vi "RT Loop - Sequence Engine.vi"(8 "error in (no error)":errorcluster, 9 "FPGA VI Reference":T1, 10 "Message Queue":refnum<queue>, 11 "Sequence Queue":refnum<queue>) -> ()   [LabVIEW 2018]
doc: "Executes the sequence sent from the main UI."
uses:
  support/Message Queue/Message Cluster.ctl
  controls/Sequence Command.ctl
  controls/Sequence Engine State.ctl
  controls/FPGA VI Reference.ctl
  controls/Control Configuration.ctl
  Globals/Global - All RT Loop Stop.vi
  <vilib>/Utility/error.llb/Error Cluster From Error Code.vi
  <vilib>/rvi/errors/niLvFpgaAdjustHostInterfaceError.vi
  <vilib>/rvi/interface/nirviReadWriteControl/nirviReadWriteControl.xnode
  NiFpgaLv.dll
  <vilib>/rvi/interface/Simulation/niFpgaSimulationCallBeginRW.vi
  support/Message Queue/Message Queue.lvlib
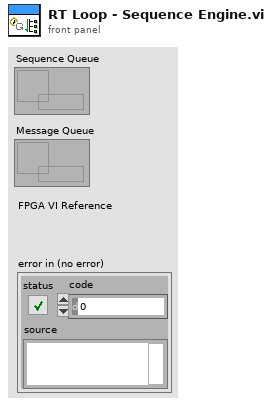
[diagram p1: front panel]
types:
  T1 = typedef "FPGA VI Reference.ctl" = refnum<k20>
  T2 = typedef "Message Queue.lvlib/Message Cluster.ctl" = cluster{"Message":string, "Message Data":variant}
  T3 = typedef "Sequence Engine State.ctl" = enum16{"Idle", "Running", "Stop", "Pause", "Resume", "Load Sequence"}
  T4 = typedef "Control Configuration.ctl" = cluster{"PID Gains":cluster{"proportional gain (Kc)":fxp<+/-,16,8>, "integral gain (Kc*Ts/Ti)":fxp<+/-,16,8>, "derivative gain (Kc*Td/Ts)":fxp<+/-,16,8>}, "Output Range":cluster{"output high":fxp<+/-,16,5>, "output low":fxp<+/-,16,5>}}
  T5 = typedef "Sequence Command.ctl" = cluster{"Sequence Engine State":T3, "Message Data":variant}
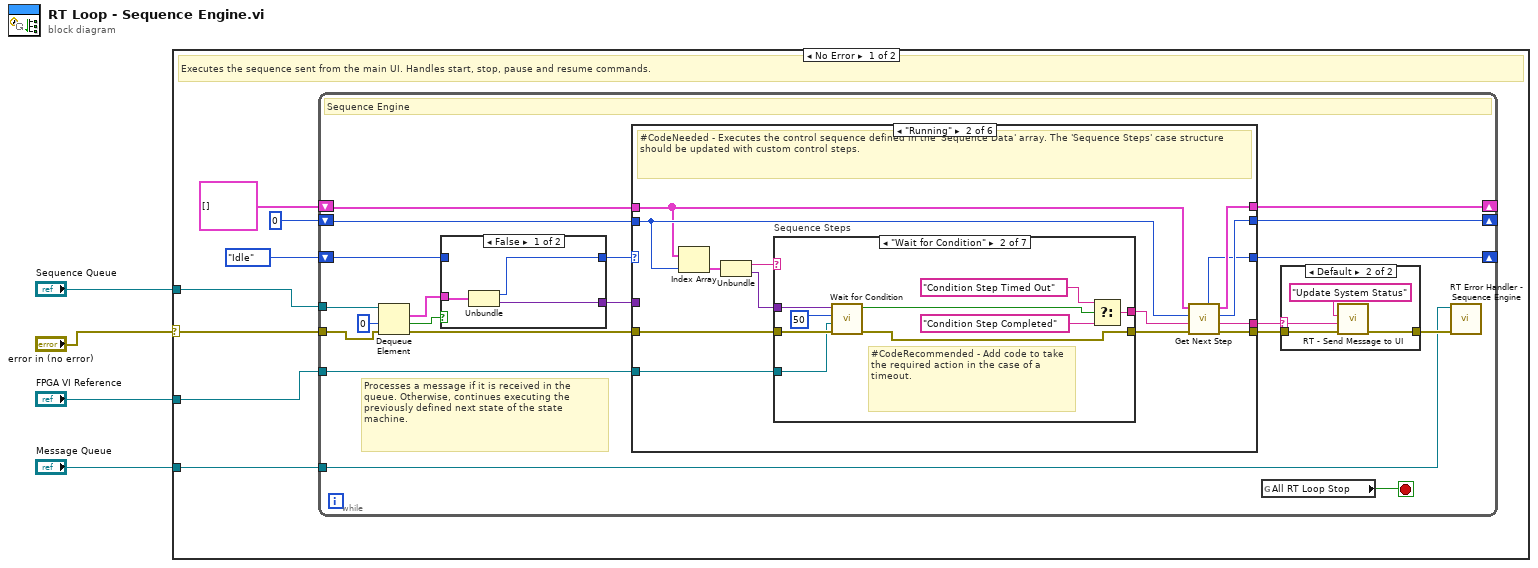
[diagram p0: block diagram]
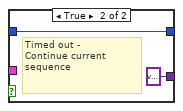
[diagram p3: hidden frame]
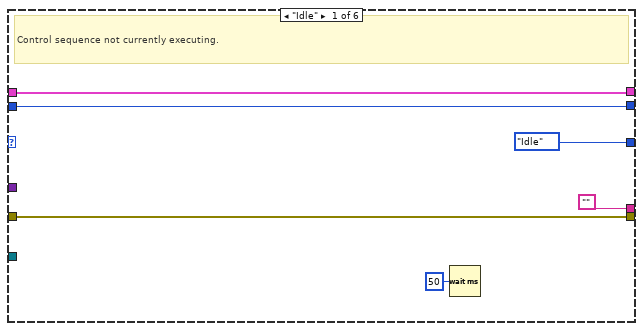
[diagram p4: hidden frame]
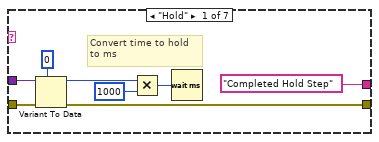
[diagram p5: hidden frame]
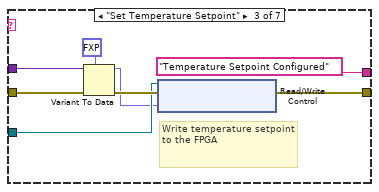
[diagram p6: hidden frame]
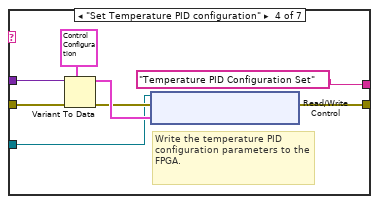
[diagram p7: hidden frame]
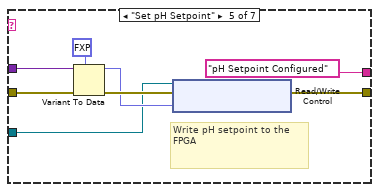
[diagram p8: hidden frame]
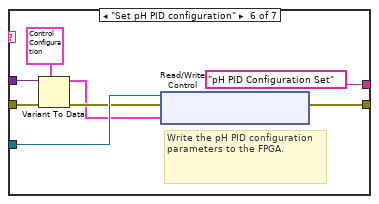
[diagram p9: hidden frame]
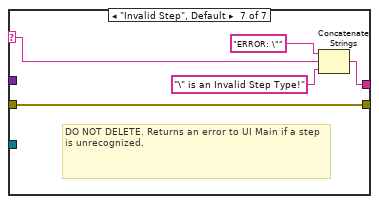
[diagram p10: hidden frame]
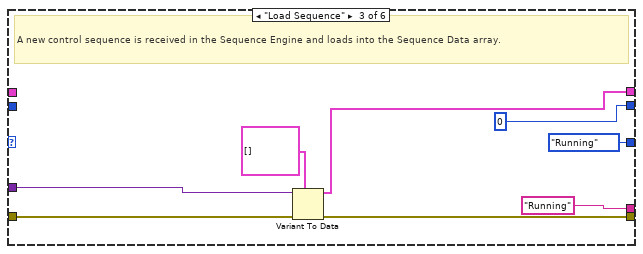
[diagram p11: hidden frame]
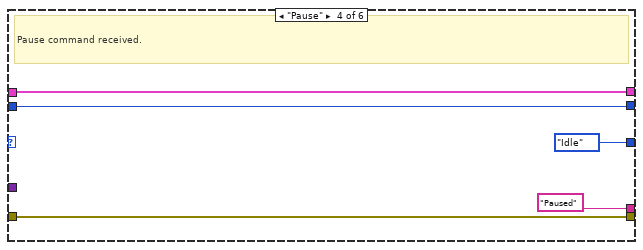
[diagram p12: hidden frame]
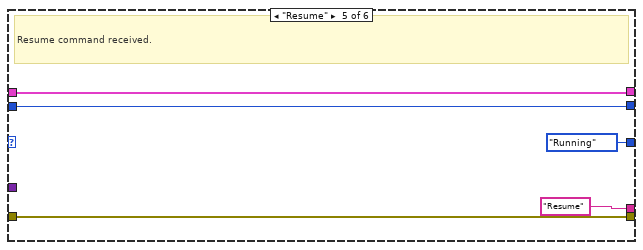
[diagram p13: hidden frame]
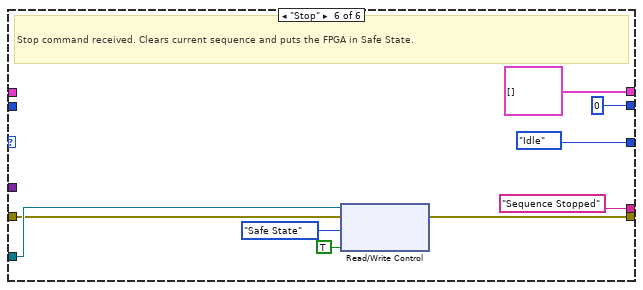
[diagram p14: hidden frame]
diagram:
  n1 = case shown="No Error" "error in (no error)" {
    selector: "error in (no error)" -> [w5 _]
    tunnel: "Message Queue" -> [w8 _]
    tunnel: "Sequence Queue" -> [w7 _]
    tunnel: "FPGA VI Reference" -> [w6 _]
    frame No Error {
      # "Executes the sequence sent from the main UI. Handles start, stop, pause and resume commands."
      n2 = while "Sequence Engine" {
        tunnel: w7 -> [w22]
        tunnel: w6 -> [w31]
        tunnel: w8 -> [w27]
        shift-right: [w28] -> _
        shift-left: Sequence_Engine_State."Idle" ("Sequence Engine State") -> [w16]
        shift-right: [w26] -> _
        shift-left: T2[] [] -> [w24]
        shift-right: [w25] -> _
        shift-left: 0 ("Current Step") -> [w23]
        tunnel: w5 -> [w21]
        stop <- w13 stop-if-true
        # "Processes a message if it is received in the queue. Otherwise, continues executing the previously defined next state of the state machine."
        # "Sequence Engine"
        n3 = Dequeue Element(queue=w22, timeout in ms (-1)=0, error in (no error)=w21) -> (element=w17:T5, timed out?=w18:bool, error out=w19:errorcluster)  [unwired: 1 out]
        n4 = case shown="False" w18 {
          tunnel: w17 -> [w39 _]
          tunnel: w16 -> [_ w41]
          tunnel: [w38 w41] -> w15
          tunnel: [w37 variant ("Message Data")] -> w14
          frame False {
            n5 = Unbundle(w39) -> ("Sequence Engine State"=w38:T3, "Message Data"=w37:variant)
          }
          frame True {
            # "Timed out - \nContinue current\nsequence"
          }
        }
        n6 = case shown="\"Running\"" w15 {
          tunnel: w19 -> [w44 w61 w122 w125 w130 w139]
          tunnel: w31 -> [_ w60 _ _ _ w141]
          tunnel: [w44 w50 w118 w125 w130 w140] -> w30
          tunnel: ["" ("f") w48 "Running" ("f") "Paused" "Resume" ("f") "Sequence Stopped"] -> w12
          tunnel: [Sequence_Engine_State."Idle" ("Sequence Engine State") w49 Sequence_Engine_State."Running" ("Sequence Engine State") Sequence_Engine_State."Idle" ("Sequence Engine State") Sequence_Engine_State."Running" ("Sequence Engine State") Sequence_Engine_State."Idle" ("Sequence Engine State")] -> w28
          tunnel: [w43 w54 w121 w128 w133 T2[] []] -> w26
          tunnel: [w42 w53 0 ("Current Step") w127 w132 0] -> w25
          tunnel: w24 -> [w43 w55 _ w128 w133 _]
          tunnel: w23 -> [w42 w56 _ w127 w132 _]
          tunnel: w14 -> [_ _ w123 _ _ _]
          frame "Idle" {
            # "Control sequence not currently executing."
            n7 = Wait (ms)(milliseconds to wait=u32 50) -> ()  [unwired: 1 out]
          }
          frame "Running" {
            # "#CodeNeeded - Executes the control sequence defined in the 'Sequence Data' array. The 'Sequence Steps' case structure should be updated with custom control steps."
            n8 = Index Array(array=w55, index=w56) -> (element=w59:T2)
            n9 = Unbundle(w59) -> ("Message"=w58:string, "Message Data"=w57:variant)
            n10 = case "Sequence Steps" shown="\"Wait for Condition\"" w58 {
              selector: w58 -> [_ _ _ _ _ _ w111]
              tunnel: w61 -> [w68 w78 w84 w91 w98 w109 w115]
              tunnel: w60 -> [_ w72 w85 w90 w97 w110 _]
              tunnel: [w64 w77 w83 w89 w99 w105 w115] -> w51
              tunnel: ["Completed Hold Step" w74 "Temperature Setpoint Configured" "Temperature PID Configuration Set" "pH Setpoint Configured" "pH PID Configuration Set" w113] -> w52
              tunnel: w57 -> [w62 w71 w79 w87 w95 w103 _]
              frame "Hold" {
                # "Convert time to hold to ms"
                n11 = Variant To Data(error in=w68, type=u32 0, Variant=w62) -> (data=w66:u32, error out=w64:errorcluster)
                n12 = Multiply(x=w66, y=u32 1000) -> (x*y=w65:u32)
                n13 = Wait (ms)(milliseconds to wait=w65) -> ()  [unwired: 1 out]
              }
              frame "Wait for Condition" {
                # "#CodeRecommended - Add code to take the required action in the case of a timeout."
                n14 = call "Wait for Condition.vi"("error in (no error)"=w78, "FPGA Refnum in"=w72, "Condition checking interval"=u32 50, "Message Data"=w71) -> ("error out"=w77:errorcluster, "Timeout?"=w76:bool)  [unwired: 6 in]
                n15 = Select(t="Condition Step Timed Out", s=w76, f="Condition Step Completed") -> (s? t:f=w74:string)
              }
              frame "Set Temperature Setpoint" {
                # "Write temperature setpoint to the FPGA"
                n16 = Variant To Data(error in=w84, type=fxp<+,1,1> 0.0, Variant=w79) -> (data=w81:fxp<+,1,1>, error out=w86:errorcluster)
                n17 = xnode "Read/Write Control"("FPGA VI Reference In"=w85, "error in"=w86, "Channel 1 Setpoint"=w81) -> ("error out"=w83:errorcluster)  [unwired: 1 out]
              }
              frame "Set Temperature PID configuration" {
                # "Write the temperature PID configuration parameters to the FPGA."
                n18 = Variant To Data(error in=w91, type=T4 {"PID Gains"={"proportional gain (Kc)"=0.0, "integral gain (Kc*Ts/Ti)"=0.0, "derivative gain (Kc*Td/Ts)"=0.0}, "Output Range"={"output high"=0.0, "output low"=0.0}} ("Control Configuration"), Variant=w87) -> (data=w94:T4, error out=w92:errorcluster)
                n19 = xnode "Read/Write Control"("FPGA VI Reference In"=w90, "error in"=w92, "Channel 1 Configuration"=w94) -> ("error out"=w89:errorcluster)  [unwired: 1 out]
              }
              frame "Set pH Setpoint" {
                # "Write pH setpoint to the FPGA"
                n20 = Variant To Data(error in=w98, type=fxp<+,1,1> 0.0, Variant=w95) -> (data=w100:fxp<+,1,1>, error out=w102:errorcluster)
                n21 = xnode "Read/Write Control"("FPGA VI Reference In"=w97, "error in"=w102, "Channel 0 Setpoint"=w100) -> ("error out"=w99:errorcluster)  [unwired: 1 out]
              }
              frame "Set pH PID configuration" {
                # "Write the pH PID configuration parameters to the FPGA."
                n22 = Variant To Data(error in=w109, type=T4 {"PID Gains"={"proportional gain (Kc)"=0.0, "integral gain (Kc*Ts/Ti)"=0.0, "derivative gain (Kc*Td/Ts)"=0.0}, "Output Range"={"output high"=0.0, "output low"=0.0}} ("Control Configuration"), Variant=w103) -> (data=w106:T4, error out=w108:errorcluster)
                n23 = xnode "Read/Write Control"("FPGA VI Reference In"=w110, "error in"=w108, "Channel 0 Configuration"=w106) -> ("error out"=w105:errorcluster)  [unwired: 1 out]
              }
              frame "Invalid Step", Default {
                # "DO NOT DELETE. Returns an error to UI Main if a step is unrecognized."
                n24 = Concatenate Strings("ERROR: \"" ("string"), w111, "\" is an Invalid Step Type!" ("t")) -> (w113:string)
              }
            }
            n25 = call "Get Next Step.vi"("error in (no error)"=w51, "Status Text In"=w52, "Current Step in"=w56, "Sequence In"=w55) -> ("error out"=w50:errorcluster, "Status Text Out"=w48:string, "Current Step out"=w53:i32, "Sequence Out"=w54:T2[], "Sequence Engine State"=w49:T3)  [unwired: 3 in]
          }
          frame "Load Sequence" {
            # "A new control sequence is received in the Sequence Engine and loads into the Sequence Data array."
            n26 = Variant To Data(error in=w122, type=T2[] [], Variant=w123) -> (data=w121:T2[], error out=w118:errorcluster)
          }
          frame "Pause" {
            # "Pause command received."
          }
          frame "Resume" {
            # "Resume command received."
          }
          frame "Stop" {
            # "Stop command received. Clears current sequence and puts the FPGA in Safe State."
            n27 = xnode "Read/Write Control"("FPGA VI Reference In"=w141, "error in"=w139, "New State"=enum16{"Safe State", "Control (PID)"}."Safe State", "Change State"=TRUE) -> ("error out"=w140:errorcluster)  [unwired: 1 out]
          }
        }
        n28 = global read "Global - All RT Loop Stop.vi" "All RT Loop Stop"() -> (w13:bool)
        n29 = case shown="Default" w12 {
          selector: w12 -> [_ w33]
          tunnel: w30 -> [w32 w36]
          tunnel: [w32 w34] -> w29
          frame "" {
            # "Blank. Send nothing."
          }
          frame Default {
            n30 = call "RT - Send Message to UI.vi"("error in (no error)"=w36, "Message Data"=w33, "Message"="Update System Status") -> ("error out"=w34:errorcluster)  [unwired: 8 in]
          }
        }
        n31 = call "RT Error Handler - Sequence Engine.vi"("error in (no error)"=w29, "Message Queue"=w27) -> ()  [unwired: 9 in, 1 out]
      }
    }
    frame Error {
      # "Input Error. Do nothing."
    }
  }
